vi "saving.vi"(1 "error in (no error)":errorcluster, 2 "Array in":dbl[](array[numeric])) -> (0 "error out":errorcluster)   [LabVIEW 2021]
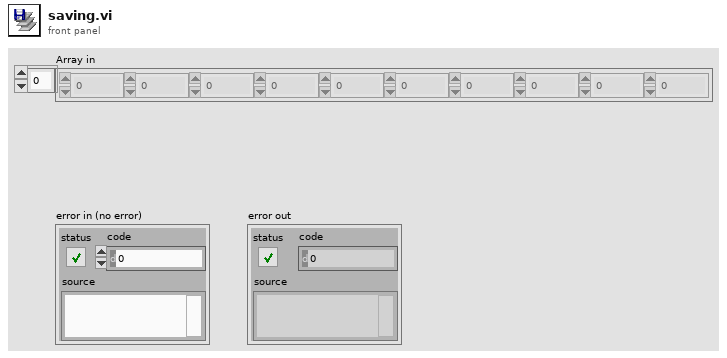
[diagram p1: front panel]
types:
  T1 = enum16{"open", "replace", "create", "open or create", "replace or create", "replace or create with confirmation"}
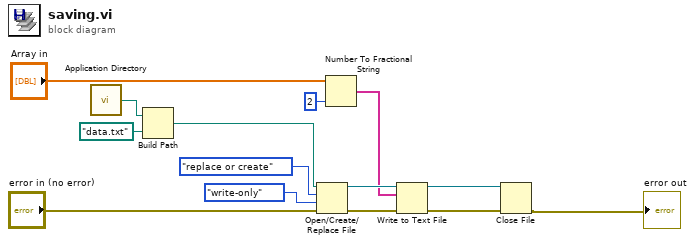
[diagram p0: block diagram]
diagram:
  n1 = call <vilib>:"Application Directory.vi"() -> ("Application Directory"=w7:path)
  n2 = Build Path(base path=w7, name or relative path=path "data.txt") -> (appended path=w5:path)
  n3 = Open/Create/Replace File(file path (use dialog)=w5, error in="error in (no error)", operation (0:open)=T1."replace or create", access (0:read/write)=enum16{"read/write", "read-only", "write-only"}."write-only") -> (refnum out=w13:refnum<file>, error out=w8:errorcluster)  [unwired: 2 in, 1 out]
  n4 = Number To Fractional String(number="Array in", precision (6)=i16 2) -> (F-format string=w12:string[])  [unwired: 2 in]
  n5 = Write to Text File(file (use dialog)=w13, text=w12, error in=w8) -> (refnum out=w11:refnum<file>, error out=w9:errorcluster)  [unwired: 1 in, 1 out]
  n6 = Close File(refnum=w11, error in=w9) -> (error out=→"error out":errorcluster)  [unwired: 1 out]
